vi "pwrite serial.vi"(6 "timoccur":i32, 7 "timeo":i32, 9 "bsize":i32, 10 "buf":i8, 11 "h":u32) -> (2 "buf out":i8, 3 "function return":i32, 4 "timoccur out":i32)   [LabVIEW 2010, in "libcommon_serial.lvlib"]
doc: "int pwrite_serial(pserial_handle_t h, char*buf,int bsize,int timeo,int*timoccur);"
uses:
  <userlib>/libcommon_serial/libcommon_serial.lvlib
  <userlib>/libcommon_serial/libcommon_serial.so
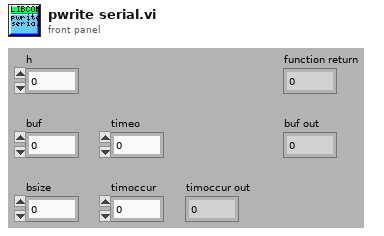
[diagram p1: front panel]
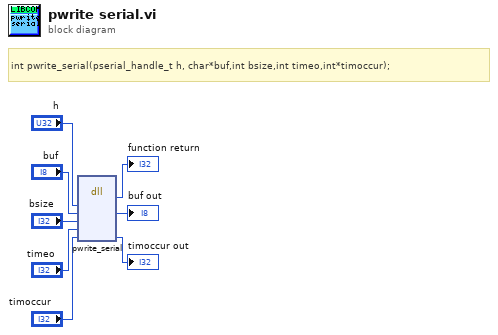
[diagram p0: block diagram]
diagram:
  # "int pwrite_serial(pserial_handle_t h, char*buf,int bsize,int timeo,int*timoccur);"
  n1 = dll-call lib="usr/local/natinst/LabVIEW-2010/user.lib/libcommon_serial/libcommon_serial.*" fn="pwrite_serial"("h"="h", "buf"="buf", "bsize"="bsize", "timeo"="timeo", "timoccur"="timoccur") -> (→"function return":i32, "buf"=→"buf out":i8, "timoccur"=→"timoccur out":i32)  [unwired: 6 in, 2 out]
